vi "Warning Max Level.vi"(11 "数组":enum16{"", "Ⅰ", "Ⅱ", "Ⅲ", "Ⅳ", "Ⅴ"}[](array[ring])) -> (3 "level":enum16{"", "Ⅰ", "Ⅱ", "Ⅲ", "Ⅳ", "Ⅴ"}(ring))   [LabVIEW 2020]
uses:
  ce8f07c8-2037-44c6-97e1-ce9ba6b562ba.vi
  26bdfb62-dda1-4d6e-b4c4-5ff4010fd95f.vi
  <vilib>/Comparison/Less/Less Functor/Less Functor.lvclass
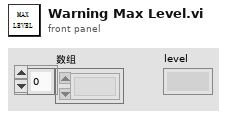
[diagram p1: front panel]
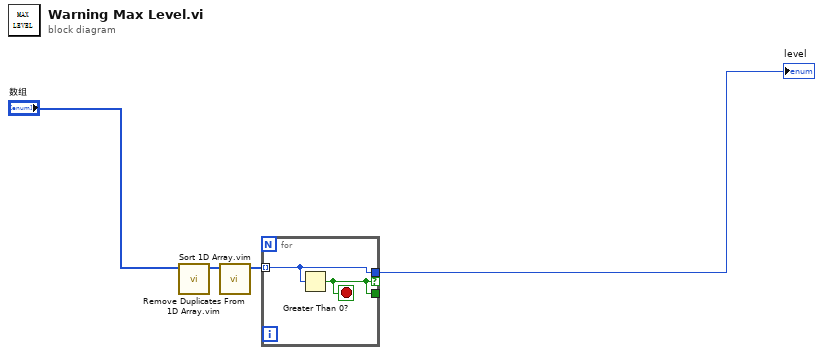
[diagram p0: block diagram]
diagram:
  n1 = call "Remove Duplicates From 1D Array.vim"("array"="数组") -> ("array with duplicates removed"=w2:enum16{"", "Ⅰ", "Ⅱ", "Ⅲ", "Ⅳ", "Ⅴ"}[])  [unwired: 10 in]
  n2 = call "Sort 1D Array.vim"("unsorted array"=w2) -> ("sorted array"=w3:enum16{"", "Ⅰ", "Ⅱ", "Ⅲ", "Ⅳ", "Ⅴ"}[])  [unwired: 10 in]
  n3 = for {
    tunnel: w3 -> [w6] mode=indexing
    tunnel: [w6] -> w4 if=w5
    tunnel: [w5] -> _
    stop <- w5 stop-if-true
    n4 = Greater Than 0?(x=w6) -> (x > 0?=w5:bool)
  }
  "level" <- w4
